vi "NodMcu interlink labview_5.vi"() -> ()   [LabVIEW 2015]
panel:
  in  "?":enum32{"Page 1", "Page 2"}(tab)
  in  "Manual":bool
  in  "Automatic":bool
  out "Rfid Detector":string
  in  "stop":bool
  in  "IP":string
  out "?":bool
  # "Pardeep Kumar"
  # "Switches"
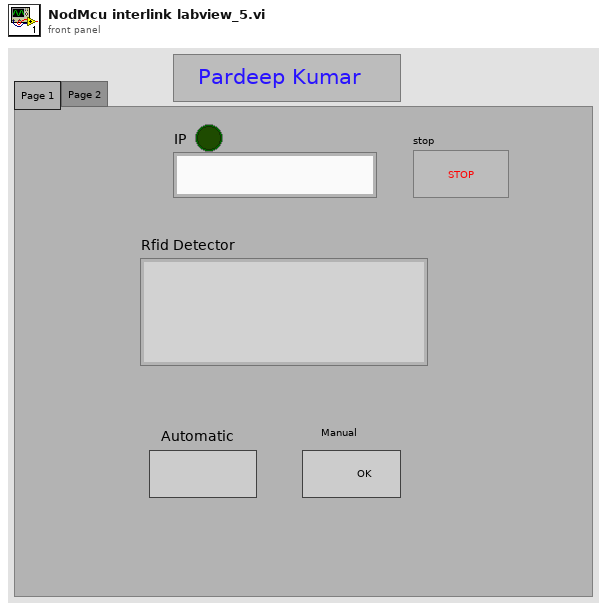
[diagram p1: front panel]
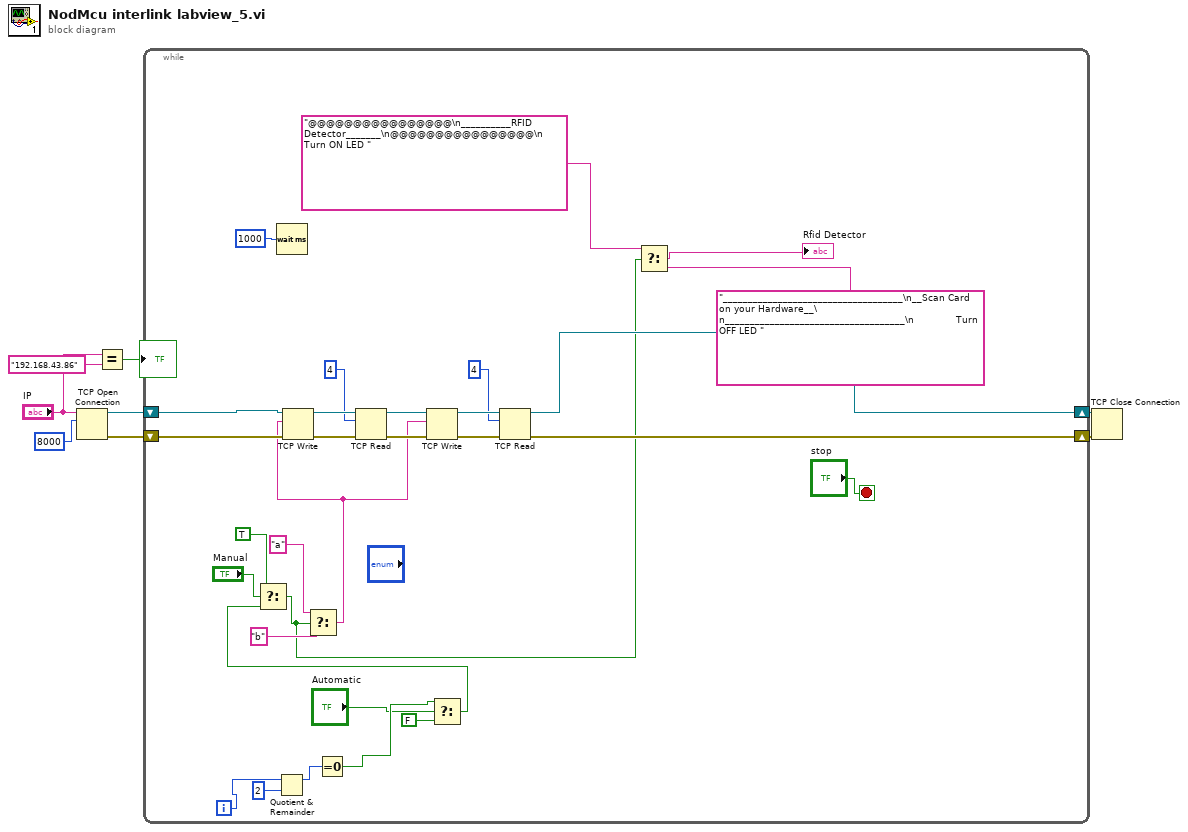
[diagram p0: block diagram]
diagram:
  n1 = TCP Open Connection(address="IP", remote port or service name=u16 8000) -> (connection ID=w7:refnum<k5>, error out=w6:errorcluster)  [unwired: 3 in]
  n2 = Equal?(x="IP", y="192.168.43.86") -> (x = y?=→"?":bool)
  n3 = while {
    shift-right: [w29] -> w5
    shift-left: w7 -> [w38]
    shift-right: [w26] -> w4
    shift-left: w6 -> [w37]
    i -> [w19]
    stop <- "stop" stop-if-true
    n4 = Wait (ms)(milliseconds to wait=u32 1000) -> ()  [unwired: 1 out]
    n5 = Quotient & Remainder(x=w19, y=2) -> (x-y*floor(x/y)=w17:i32)  [unwired: 1 out]
    n6 = Equal To 0?(x=w17) -> (x = 0?=w15:bool)
    n7 = Select(t=w15, s="Automatic", f=FALSE) -> (s? t:f=w10:bool)
    n8 = Select(t=TRUE ("f"), s="Manual", f=w10) -> (s? t:f=w9:bool)
    n9 = Select(t="a", s=w9, f="b" ("data in")) -> (s? t:f=w24:string)
    n10 = TCP Write(connection ID=w38, data in=w24, error in (no error)=w37) -> (connection ID out=w36:refnum<k5>, error out=w35:errorcluster)  [unwired: 1 in, 1 out]
    n11 = TCP Read(connection ID=w36, bytes to read=4, error in (no error)=w35) -> (connection ID out=w31:refnum<k5>, error out=w28:errorcluster)  [unwired: 2 in, 1 out]
    n12 = TCP Write(connection ID=w31, data in=w24, error in (no error)=w28) -> (connection ID out=w30:refnum<k5>, error out=w27:errorcluster)  [unwired: 1 in, 1 out]
    n13 = TCP Read(connection ID=w30, bytes to read=4, error in (no error)=w27) -> (connection ID out=w29:refnum<k5>, error out=w26:errorcluster)  [unwired: 2 in, 1 out]
    n14 = Select(t="@@@@@@@@@@@@@@@@\n__________RFID Detector_______\n@@@@@@@@@@@@@@@@\n               Turn ON LED ", s=w9, f="____________________________________\n__Scan Card on your Hardware__\n____________________________________\n              Turn OFF LED ") -> (s? t:f=→"Rfid Detector":string)
  }
  n15 = TCP Close Connection(connection ID=w5, error in (no error)=w4) -> ()  [unwired: 1 in, 2 out]
